vi "TCP Write.vi"(7 "Timeout (2000)":i32=2000, 8 "Error In":errorcluster, 10 "Packet":string, 11 "LINX Decice Config":T1) -> (0 "Error Out":errorcluster, 3 "LINX Decice Config":T1)   [LabVIEW 2020, in "Device.lvlib"]
uses:
  Device.lvlib
  Type Defs/LINX Device Config.ctl
  Type Defs/Interface.ctl
  Type Defs/TCP Config.ctl
  Type Defs/Channels.ctl
  Type Defs/Error Type.ctl
  LMH-LINX.lvlib
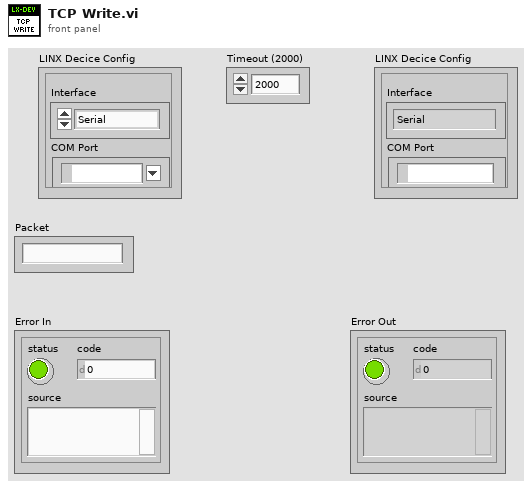
[diagram p1: front panel]
types:
  T1 = typedef "Device.lvlib/LINX Device Config.ctl" = cluster{"Interface":T2, "COM Port":refnum<visa-resource-name>, "TCP Configuration":T3, "Device Family":u8, "Device ID":u8, "Device Name":string, "TCP Ref":refnum<k5>, "Channels":T4}
  T2 = typedef "LMH-LINX.lvlib/Interface.ctl" = enum16{"Serial", "TCP"}
  T3 = typedef "Device.lvlib/TCP Config.ctl" = cluster{"IP Address":string, "Port":u16}
  T4 = typedef "LMH-LINX.lvlib/Channels.ctl" = cluster{"DI":u8[], "DO":u8[], "AI":u8[], "AO":u8[], "PWM":u8[], "QE":u8[], "UART":u8[], "I2C 2":u8[], "SPI":u8[], "CAN":u8[], "Servo":u8[], "AI Ref (V)":dbl, "AI Resolution (Bits)":u8, "AO Ref (V)":dbl, "AO Resolution (Bits)":u8}
  T5 = typedef "LMH-LINX.lvlib/Error Type.ctl" = enum16{"Unknown", "Timeout", "Corrupt Return Packet", "Unable To Connect", "Command Not Supported", "Channel DNE", "Invalid COM Config", "Firmware Version Mismatch", "myRIO Support", "CMD Specific Error", "Local IO Not Supported"}
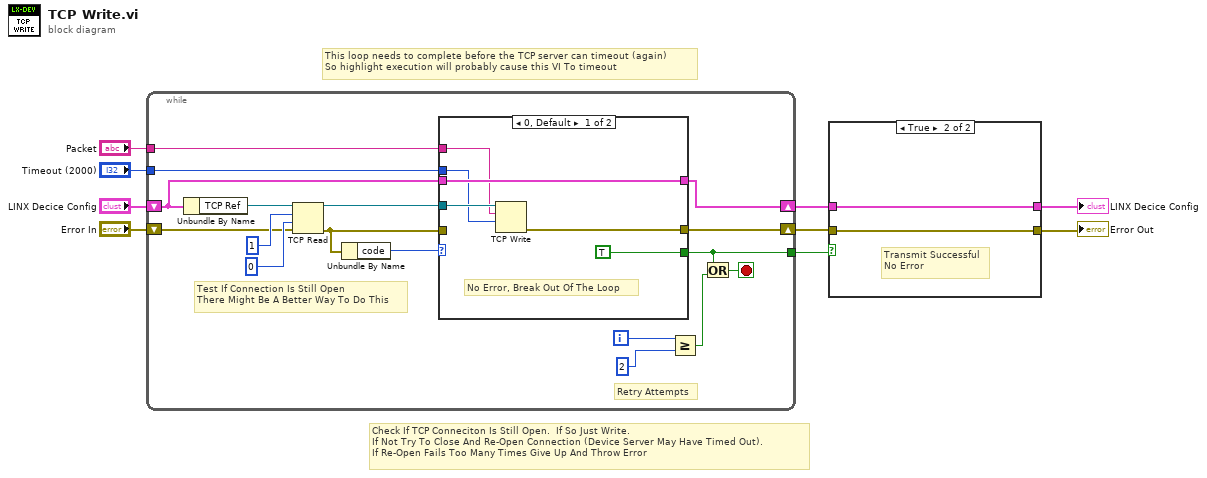
[diagram p0: block diagram]
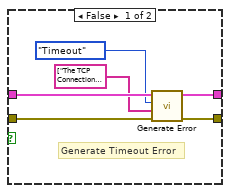
[diagram p2: hidden frame]
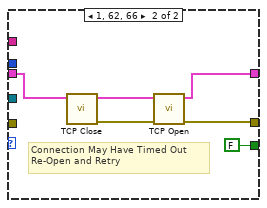
[diagram p3: hidden frame]
diagram:
  # "This loop needs to complete before the TCP server can timeout (again)\nSo highlight execution will probably cause this VI To timeout"
  # "Check If TCP Conneciton Is Still Open.  If So Just Write.\nIf Not Try To Close And Re-Open Connection (Device Server May Have Timed Out).\nIf Re-Open Fails Too Many Times Give Up And Throw Error"
  n1 = while {
    tunnel: "Packet" -> [w11]
    tunnel: "Timeout (2000)" -> [w10]
    tunnel: [w21] -> w4
    shift-right: [w26] -> w5
    shift-left: "Error In" -> [w16]
    shift-right: [w20] -> w3
    shift-left: "LINX Decice Config" -> [w19]
    i -> [w24]
    stop <- w25 stop-if-true
    # "Retry Attempts"
    # "Test If Connection Is Still Open\nThere Might Be A Better Way To Do This"
    n2 = Unbundle By Name(w19) -> ("TCP Ref"=w15:refnum<k5>)
    n3 = TCP Read(connection ID=w15, bytes to read=1, error in (no error)=w16, 9:0 ("timeout ms (25000)")) -> (connection ID out=w12:refnum<k5>, error out=w13:errorcluster)  [unwired: 1 in, 1 out]
    n4 = Unbundle By Name(w13) -> ("code"=w14:i32)
    n5 = case shown="0, Default" w14 {
      tunnel: w19 -> [w31 w36]
      tunnel: [w30 w33] -> w26
      tunnel: [TRUE FALSE] -> w21
      tunnel: [w31 w37] -> w20
      tunnel: w13 -> [_ _]
      tunnel: w12 -> [w29 _]
      tunnel: w11 -> [w28 _]
      tunnel: w10 -> [w27 _]
      frame 0, Default {
        # "No Error, Break Out Of The Loop"
        n6 = TCP Write(connection ID=w29, data in=w28, 9:w27) -> (error out=w30:errorcluster)  [unwired: 1 in, 2 out]
      }
      frame 1, 62, 66 {
        # "Connection May Have Timed Out\nRe-Open and Retry"
        n7 = call "TCP Close.vi"("LINX Decice Config"=w36) -> ("Error Out"=w34:errorcluster, "LINX Decice Config"=w35:T1)  [unwired: 9 in]
        n8 = call "TCP Open.vi"("Error In"=w34, "LINX Device Config"=w35) -> ("Error Out"=w33:errorcluster, "LINX Device Config"=w37:T1)  [unwired: 8 in]
      }
    }
    n9 = Greater Or Equal?(x=w24, y=2) -> (x >= y?=w22:bool)
    n10 = Or(x=w21, y=w22) -> (x .or. y?=w25:bool)
  }
  n11 = case shown="True" w4 {
    tunnel: [w44 w46] -> w6
    tunnel: w5 -> [w43 w46]
    tunnel: w3 -> [w42 w45]
    tunnel: [w39 w45] -> w1
    frame False {
      # "Generate Timeout Error"
      n12 = call "Generate Error.vi"("Error In"=w43, "Arguments"=string[] ["The TCP Connection Was Refused."], "Error Type"=Error_Type."Timeout", "LINX Device Config"=w42) -> ("Error Out"=w44:errorcluster, "Dup LINX Device Config"=w39:T1)  [unwired: 6 in]
    }
    frame True {
      # "Transmit Successful\nNo Error"
    }
  }
  "Error Out" <- w6
  "LINX Decice Config" <- w1
